vi "SUNSoftwareBinCheckReceivedQty.vi"() -> ()   [LabVIEW 2012]
uses:
  <vilib>/addons/database/Auxilliary.llb/DB Tools Cursor Type.ctl
  <vilib>/Utility/NIReport.llb/NI_report.lvclass
  <vilib>/addons/database/Connection.llb/DB Tools Open Connec (Path).vi
  <vilib>/addons/database/Connection.llb/Conn Execute.vi
  <vilib>/addons/database/Recordset.llb/Rec Fetch Recordset Data (R).vi
  <vilib>/addons/database/Recordset.llb/Rec Destroy - Connection.vi
  <vilib>/addons/database/Recordset.llb/Rec Fetch Integer Data (R).vi
  <vilib>/Utility/NIReport.llb/Append Text Table to Report (wrap).vi
  <vilib>/addons/database/_DB Variant To Data/Database Variant To Data.xnode
  <vilib>/addons/database/NI_Database_API.lvlib
  <vilib>/Utility/NIReport.llb/Excel/NI_Excel.lvclass
panel:
  out "recordset data":variant[][](array[variant])
  out "data":string
  out "appended array":string[](array[string])
  out "concatenated string":string
  in  "Report Template":path=path "O:/Monitor/Report/MSTsoftBin.xls"
  out "Row Headers":string[](array[string])
  out "error out 2":errorcluster
  out "error out":errorcluster
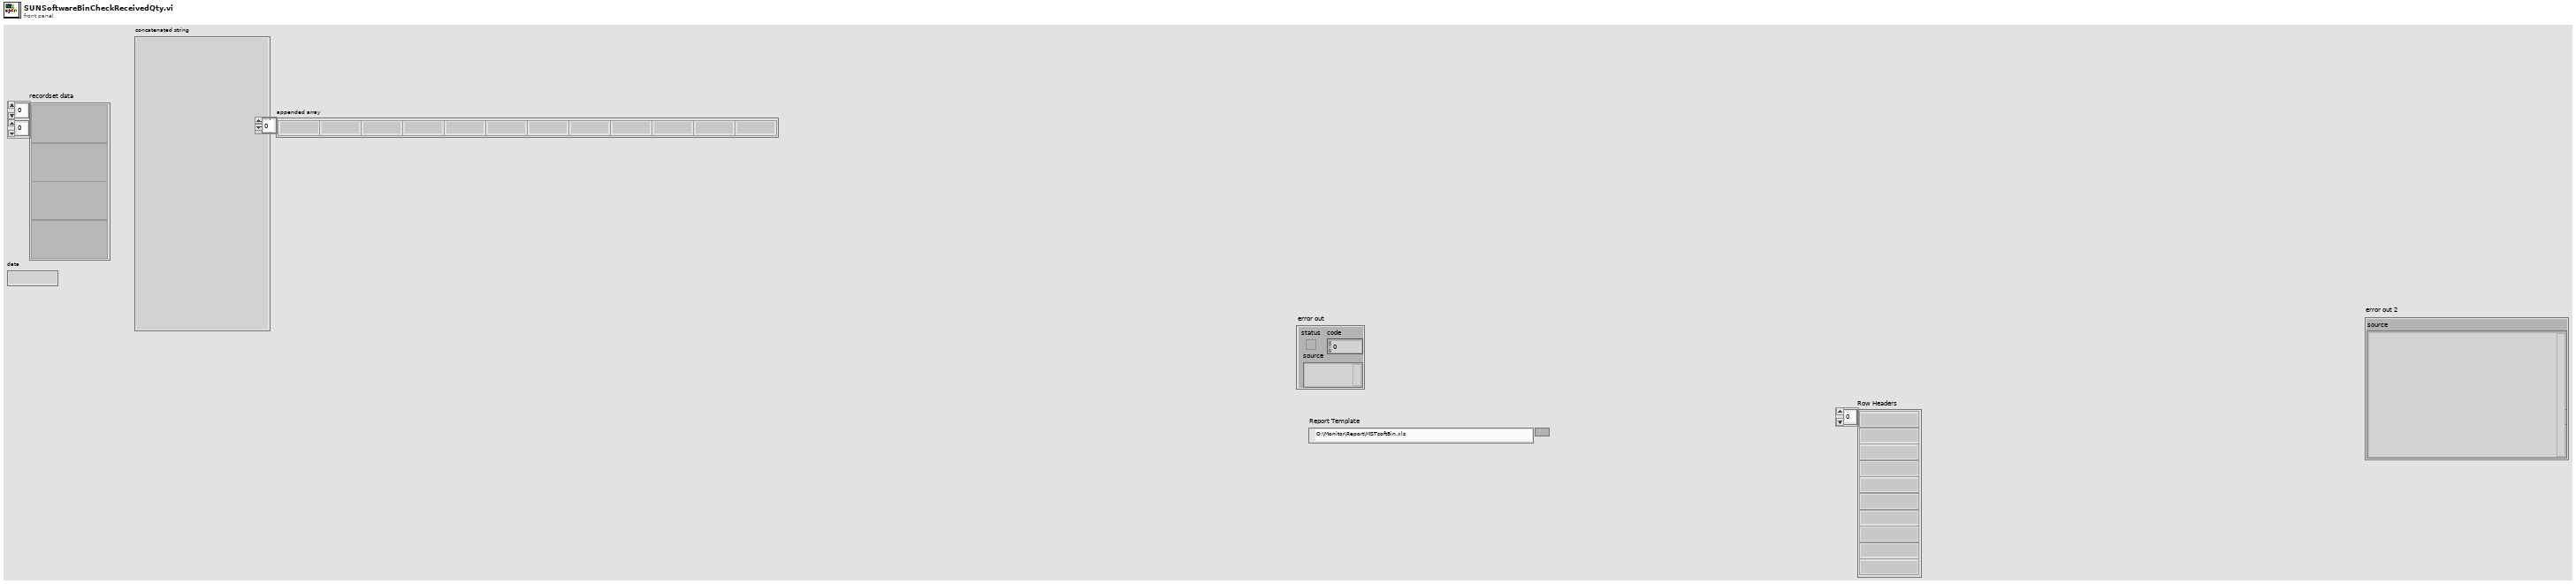
[diagram p1: front panel]
types:
  T1 = typedef "NI_Database_API.lvlib/DB Tools Cursor Type.ctl" = enum16{"forward-only", "keyset", "dynamic", "static"}
  T2 = enum16{"Standard Report", "HTML", "Word", "Excel"}
  T3 = typedef "NI_Database_API.lvlib/Conn ObjectReference.ctl" = refnum<k1>
  T4 = typedef "NI_Database_API.lvlib/Rec ObjectReference.ctl" = refnum<k1>
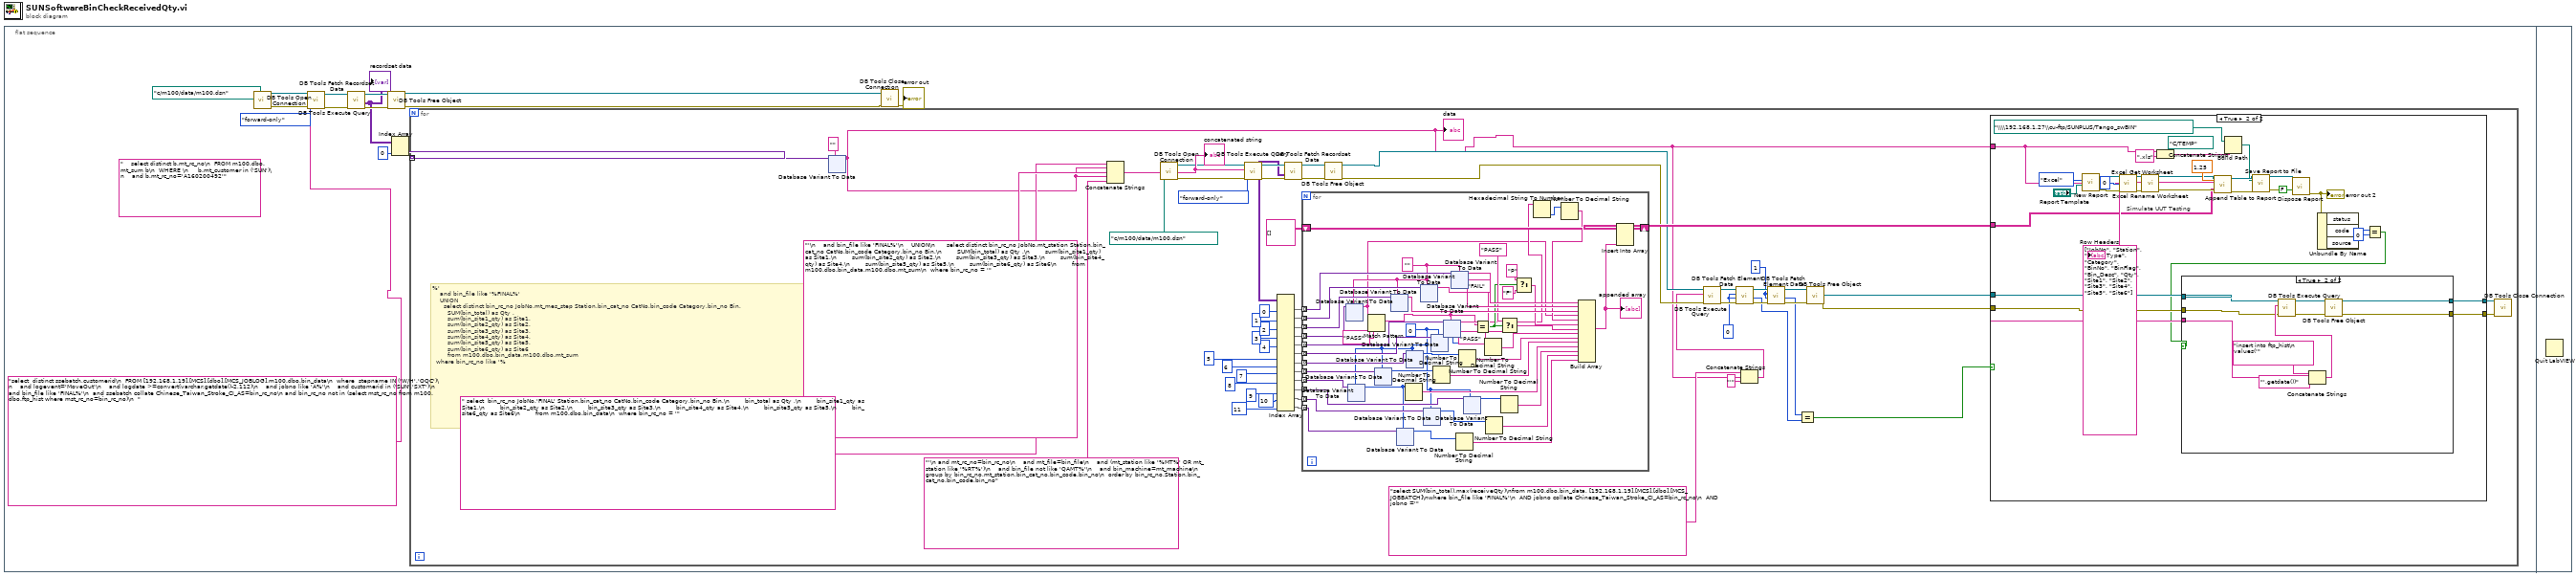
[diagram p0: block diagram]
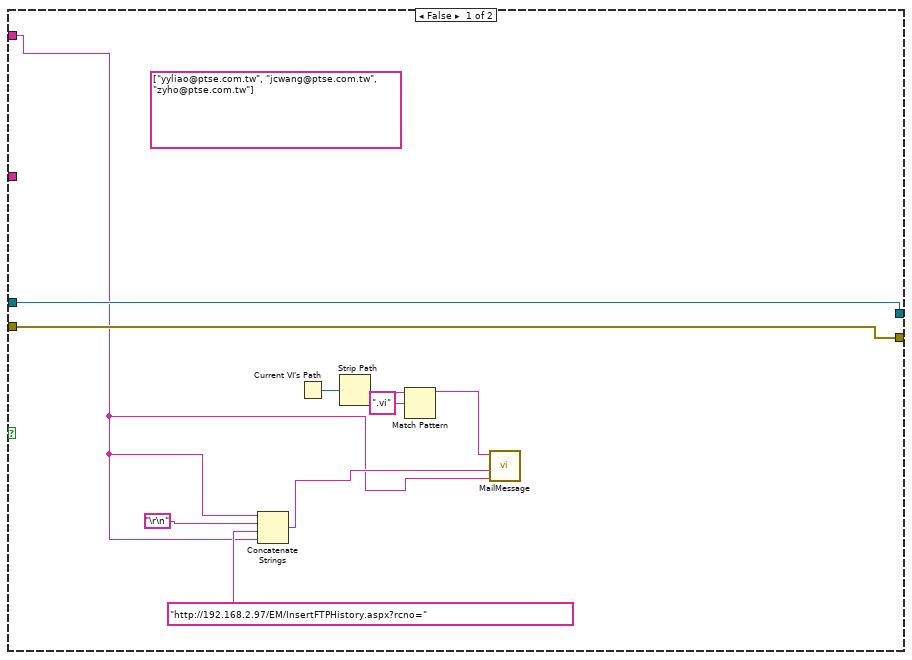
[diagram p2: hidden frame]
diagram:
  n1 = flat-sequence {
    frame #0 {
      (unwired) "    select distinct b.mt_rc_no\n  FROM m100.dbo.mt_sum b\n  WHERE \n     b.mt_customer in ('SUN')\n    and b.mt_rc_no='A160200492'" ("SQL query")
      n2 = call-poly <vilib>:"DB Tools Open Connection.vi"("connection information"=path "c:/m100/data/m100.dsn") -> ("error out"=w12:errorcluster, "connection reference"=w15:T3)  [unwired: 7 in]
      n3 = call-poly <vilib>:"DB Tools Execute Query.vi"("error in (no error)"=w12, "cursor type"=DB_Tools_Cursor_Type."forward-only", "SQL query"="select  distinct ssebatch,customerid\n  FROM [192.168.1.19].[MCS].[dbo].[MCS_JOBLOG],m100.dbo.bin_data\n  where  stepname IN ('W/H','OQC')\n    and logevent='MoveOut'\n    and logdate >=convert(varchar,getdate()-2,112)\n    and jobno like 'A%'\n    and customerid in ('SUN','SXT')\n  and bin_file like 'FINAL%'\n  and ssebatch collate Chinese_Taiwan_Stroke_CI_AS=bin_rc_no\n and bin_rc_no not in (select mst_rc_no from m100.dbo.ftp_hist where mst_rc_no=bin_rc_no)\n  ", "connection reference"=w15) -> ("error out"=w11:errorcluster, "recordset reference"=w14:T4)  [unwired: 4 in]
      n4 = call-poly <vilib>:"DB Tools Fetch Recordset Data.vi"("error in (no error)"=w11, "recordset reference"=w14) -> ("error out"=w10:errorcluster, "recordset data"=w7:variant[][], "recordset reference out"=w13:T4)  [unwired: 3 in]
      "recordset data" <- w7
      n5 = call-poly <vilib>:"DB Tools Free Object.vi"("error in (no error)"=w10, "recordset reference"=w13) -> ("error out"=w3:errorcluster, "connection reference"=w4:T3)  [unwired: 8 in]
      n6 = Index Array(array=w7, index (col)=0 ("disabled index (col)")) -> (element=w5:variant[])  [unwired: 1 in]
      n7 = for {
        tunnel: w5 -> [w77] mode=indexing
        w21 = 1
        w22 = 0
        # "%'\n    and bin_file like '%FINAL%'\n    UNION\n      select distinct bin_rc_no JobNo,mt_mes_step Station,bin_cat_no CatNo,bin_code Category,bin_no Bin,\n        SUM(bin_total) as Qty ,\n        sum(bin_site1_qty) as Site1,\n        sum(bin_site2_qty) as Site2,\n        sum(bin_site3_qty) as Site3,\n        sum(bin_site4_qty) as Site4,\n        sum(bin_site5_qty) as Site5,\n        sum(bin_site6_qty) as Site6\n        from m100.dbo.bin_data,m100.dbo.mt_sum\n  where bin_rc_no like '%"
        n8 = xnode "Database Variant To Data"("database variant"=w77, "type"="") -> ("data"=w25:string)  [unwired: 1 in, 1 out]
        "data" <- w25
        n9 = Concatenate Strings(" select  bin_rc_no JobNo,'FINAL' Station,bin_cat_no CatNo,bin_code Category,bin_no Bin,\n        bin_total as Qty ,\n        bin_site1_qty as Site1,\n        bin_site2_qty as Site2,\n        bin_site3_qty as Site3,\n        bin_site4_qty as Site4,\n        bin_site5_qty as Site5,\n        bin_site6_qty as Site6\n        from m100.dbo.bin_data\n  where bin_rc_no = '" ("string"), w25, "'\n    and bin_file like 'FINAL%'\n    UNION\n      select distinct bin_rc_no JobNo,mt_station Station,bin_cat_no CatNo,bin_code Category,bin_no Bin,\n        SUM(bin_total) as Qty ,\n        sum(bin_site1_qty) as Site1,\n        sum(bin_site2_qty) as Site2,\n        sum(bin_site3_qty) as Site3,\n        sum(bin_site4_qty) as Site4,\n        sum(bin_site5_qty) as Site5,\n        sum(bin_site6_qty) as Site6\n        from m100.dbo.bin_data,m100.dbo.mt_sum\n  where bin_rc_no = '" ("string"), w25, "'\n and mt_rc_no=bin_rc_no\n    and mt_file=bin_file\n    and (mt_station like '%MT%' OR mt_station like '%RT%')\n    and bin_file not like 'QAMT%'\n    and bin_machine=mt_machine\n  group by bin_rc_no,mt_station,bin_cat_no,bin_code,bin_no\n  order by bin_rc_no,Station,bin_cat_no,bin_code,bin_no" ("string")) -> (w68:string)
        "concatenated string" <- w68
        n10 = call-poly <vilib>:"DB Tools Open Connection.vi"("connection information"=path "c:/m100/data/m100.dsn") -> ("error out"=w39:errorcluster, "connection reference"=w40:T3)  [unwired: 7 in]
        n11 = call-poly <vilib>:"DB Tools Execute Query.vi"("error in (no error)"=w39, "cursor type"=DB_Tools_Cursor_Type."forward-only", "SQL query"=w68, "connection reference"=w40) -> ("error out"=w73:errorcluster, "recordset reference"=w75:T4)  [unwired: 4 in]
        n12 = call-poly <vilib>:"DB Tools Fetch Recordset Data.vi"("error in (no error)"=w73, "recordset reference"=w75) -> ("error out"=w72:errorcluster, "recordset data"=w67:variant[][], "recordset reference out"=w74:T4)  [unwired: 3 in]
        n13 = Index Array(array=w67, index (col) #1=0 ("disabled index (col)"), index (col) #2=1 ("index (col)"), index (col) #3=2 ("index (col)"), index (col) #4=3 ("index (col)"), index (col) #5=4 ("index (col)"), index (col) #6=5 ("index (col)"), index (col) #7=6 ("index (col)"), index (col) #8=7 ("index (col)"), index (col) #9=8 ("index (col)"), index (col) #10=9 ("index (col)"), index (col) #11=10 ("index (col)"), index (col) #12=11 ("index (col)")) -> (element #1=w56:variant[], element #2=w55:variant[], element #3=w54:variant[], element #4=w53:variant[], element #5=w52:variant[], element #6=w51:variant[], element #7=w50:variant[], element #8=w49:variant[], element #9=w48:variant[], element #10=w47:variant[], element #11=w44:variant[], element #12=w43:variant[])  [unwired: 12 in]
        n14 = for {
          tunnel: w56 -> [w177] mode=indexing
          tunnel: w55 -> [w176] mode=indexing
          tunnel: w54 -> [w175] mode=indexing
          tunnel: w53 -> [w174] mode=indexing
          tunnel: w52 -> [w173] mode=indexing
          tunnel: w51 -> [w172] mode=indexing
          tunnel: w50 -> [w171] mode=indexing
          tunnel: w49 -> [w170] mode=indexing
          tunnel: w48 -> [w169] mode=indexing
          tunnel: w47 -> [w168] mode=indexing
          tunnel: w44 -> [w159] mode=indexing
          tunnel: w43 -> [w158] mode=indexing
          shift-right: [w153] -> w41
          shift-left: string[][] [] ("array") -> [w152]
          w144 = 0
          w167 = ""
          n15 = xnode "Database Variant To Data"("database variant"=w174, "type"=w167) -> ("data"=w132:string)  [unwired: 1 in, 1 out]
          n16 = xnode "Database Variant To Data"("database variant"=w169, "type"=w144) -> ("data"=w156:i32)  [unwired: 1 in, 1 out]
          n17 = Match Pattern(string=w132, regular expression="PASS") -> (match substring=w130:string)  [unwired: 1 in, 3 out]
          n18 = xnode "Database Variant To Data"("database variant"=w170, "type"=w144) -> ("data"=w161:i32)  [unwired: 1 in, 1 out]
          n19 = xnode "Database Variant To Data"("database variant"=w175, "type"=w167) -> ("data"=w164:string)  [unwired: 1 in, 1 out]
          n20 = xnode "Database Variant To Data"("database variant"=w158, "type"=w156) -> ("data"=w157:i32)  [unwired: 1 in, 1 out]
          n21 = Number To Decimal String(number=w156) -> (decimal integer string=w148:string)  [unwired: 1 in]
          n22 = xnode "Database Variant To Data"("database variant"=w171, "type"=w144) -> ("data"=w162:i32)  [unwired: 1 in, 1 out]
          n23 = xnode "Database Variant To Data"("database variant"=w176, "type"=w167) -> ("data"=w165:string)  [unwired: 1 in, 1 out]
          n24 = xnode "Database Variant To Data"("database variant"=w159, "type"=w144) -> ("data"=w155:i32)  [unwired: 1 in, 1 out]
          n25 = xnode "Database Variant To Data"("database variant"=w172, "type"=w144) -> ("data"=w163:i32)  [unwired: 1 in, 1 out]
          n26 = Number To Decimal String(number=w161) -> (decimal integer string=w147:string)  [unwired: 1 in]
          n27 = xnode "Database Variant To Data"("database variant"=w173, "type"=w130) -> ("data"=w134:string)  [unwired: 1 in, 1 out]
          n28 = xnode "Database Variant To Data"("database variant"=w177, "type"=w167) -> ("data"=w166:string)  [unwired: 1 in, 1 out]
          n29 = Number To Decimal String(number=w157) -> (decimal integer string=w151:string)  [unwired: 1 in]
          n30 = Number To Decimal String(number=w162) -> (decimal integer string=w146:string)  [unwired: 1 in]
          n31 = xnode "Database Variant To Data"("database variant"=w168, "type"=w144) -> ("data"=w160:i32)  [unwired: 1 in, 1 out]
          n32 = Equal?(x=w130, y="PASS") -> (x = y?=w140:bool)
          n33 = Number To Decimal String(number=w163) -> (decimal integer string=w145:string)  [unwired: 1 in]
          n34 = Number To Decimal String(number=w155) -> (decimal integer string=w150:string)  [unwired: 1 in]
          n35 = Number To Decimal String(number=w160) -> (decimal integer string=w149:string)  [unwired: 1 in]
          n36 = Select(t="PASS", s=w140, f="FAIL") -> (s? t:f=w141:string)
          n37 = Select(t="P", s=w140, f="F") -> (s? t:f=w137:string)
          n38 = Hexadecimal String To Number(string=w134) -> (number=w135:u32)  [unwired: 2 in, 1 out]
          n39 = Number To Decimal String(number=w135) -> (decimal integer string=w133:string)  [unwired: 1 in]
          n40 = Build Array(w166, w165, w164, w132, w133, w137, w141, w145, w146, w147, w148, w149, w150, w151) -> (w154:string[])
          "appended array" <- w154
          n41 = Insert Into Array(array=w152, new element=w154) -> (w153:string[][])  [unwired: 2 in]
        }
        n42 = call-poly <vilib>:"DB Tools Free Object.vi"("error in (no error)"=w72, "recordset reference"=w74) -> ("error out"=w35:errorcluster, "connection reference"=w36:T3)  [unwired: 8 in]
        n43 = Concatenate Strings("select SUM(bin_total),max(receiveQty)\nfrom m100.dbo.bin_data, [192.168.1.19].[MCS].[dbo].[MCS_JOBBATCH]\nwhere bin_file like 'FINAL%'\n  AND jobno collate Chinese_Taiwan_Stroke_CI_AS=bin_rc_no\n  AND jobno ='" ("SQL query"), w25, "'" ("string")) -> (w23:string)
        n44 = call-poly <vilib>:"DB Tools Execute Query.vi"("error in (no error)"=w35, "SQL query"=w23, "connection reference"=w36) -> ("error out"=w33:errorcluster, "recordset reference"=w34:T4)  [unwired: 5 in]
        n45 = call-poly <vilib>:"DB Tools Fetch Element Data.vi"("error in (no error)"=w33, "type"=w22, "column index"=w22, "recordset reference"=w34) -> ("error out"=w31:errorcluster, "data"=w19:i32, "recordset reference out"=w32:T4)  [unwired: 3 in]
        n46 = call-poly <vilib>:"DB Tools Fetch Element Data.vi"("error in (no error)"=w31, "type"=w21, "column index"=w21, "recordset reference"=w32) -> ("error out"=w29:errorcluster, "data"=w20:i32, "recordset reference out"=w30:T4)  [unwired: 3 in]
        n47 = Equal?(x=w20, y=w19) -> (x = y?=w16:bool)
        n48 = call-poly <vilib>:"DB Tools Free Object.vi"("error in (no error)"=w29, "recordset reference"=w30) -> ("error out"=w27:errorcluster, "connection reference"=w28:T3)  [unwired: 8 in]
        n49 = case shown="True" w16 {
          tunnel: w41 -> [_ w106]
          tunnel: w28 -> [w87 w93]
          tunnel: w27 -> [w86 w92]
          tunnel: w25 -> [w78 w91]
          tunnel: [w87 w89] -> w18
          tunnel: [w86 w88] -> w17
          frame False {
            (unwired) string[] ["yyliao@ptse.com.tw", "jcwang@ptse.com.tw", "zyho@ptse.com.tw"] ("recipients")
            n50 = Concatenate Strings(w78, "\r\n", "http://192.168.2.97/EM/InsertFTPHistory.aspx?rcno=" ("string"), w78) -> (w79:string)
            n51 = Current VI's Path() -> (path=w83:path)
            n52 = Strip Path(path=w83) -> (name=w82:string)  [unwired: 1 out]
            n53 = Match Pattern(string=w82, regular expression=".vi") -> (before substring=w80:string)  [unwired: 1 in, 3 out]
            n54 = call "MailMessage.vi"("AddSubject"=w78, "message"=w79, "program"=w80) -> ()  [unwired: 9 in]
          }
          frame True {
            (unwired) path "C:/TEMP" ("base path")
            # "Simulate UUT Testing"
            n55 = call <vilib>:"New Report.vi"("report type"=T2."Excel" ("Report Type"), "template (empty)"="Report Template") -> ("report out"=w113:refnum<class "NI_report.lvclass">, "error out"=w112:errorcluster)  [unwired: 12 in]
            n56 = call <vilib>:"Excel Get Worksheet.vi"("report in"=w113, "worksheet index (0)"=0, "error in (no error)"=w112) -> ("report out"=w110:refnum<class "NI_report.lvclass">, "error out"=w108:errorcluster)  [unwired: 11 in]
            n57 = call <vilib>:"Excel Rename Worksheet.vi"("report in"=w110, "worksheet name (\"\")"=w91, "error in (no error)"=w108) -> ("report out"=w109:refnum<class "NI_report.lvclass">, "error out"=w107:errorcluster)  [unwired: 11 in]
            n58 = Concatenate Strings(w91, ".xls" ("string")) -> (w99:string)
            n59 = call-poly <vilib>:"Append Table to Report.vi"("report in"=w109, "column width (1)"=1.25, "column headers"=string[] ["JobNo", "Station", "CatNo Type", "Category", "BinNo", "BinFlag", "Bin_Desc", "Qty", "Site1", "Site2", "Site3", "Site4", "Site5", "Site6"] ("row headers"), "text data"=w106, "error in (no error)"=w107) -> ("report out"=w102:refnum<class "NI_report.lvclass">, "error out"=w101:errorcluster)  [unwired: 7 in, 2 out]
            n60 = Build Path(base path=path "\\\\192.168.1.27\\cu-ftp/SUNPLUS/Tango_swBIN", name or relative path=w99) -> (appended path=w98:path)
            n61 = call-dynamic "Save Report to File.vi"("report in"=w102, "report file path"=w98, "error in (no error)"=w101) -> ("report out"=w104:refnum<class "NI_report.lvclass">, "error out"=w103:errorcluster)  [unwired: 11 in]
            n62 = call-dynamic "Dispose Report.vi"("report in"=w104, "save changes? (F)"=FALSE, "error in (no error)"=w103) -> ("error out"=w97:errorcluster)  [unwired: 12 in]
            "error out 2" <- w97
            n63 = Unbundle By Name(w97) -> ("code"=w96:i32)  [unwired: 2 out]
            n64 = Equal?(x=w96, y=0) -> (x = y?=w90:bool)
            n65 = case shown="True" w90 {
              tunnel: w93 -> [w119 w129]
              tunnel: w91 -> [_ w127]
              tunnel: [w119 w122] -> w89
              tunnel: [w118 w121] -> w88
              tunnel: w92 -> [w118 w120]
              frame False {
              }
              frame True {
                n66 = Concatenate Strings("insert into ftp_hist\n values('" ("string"), w127, "',getdate())" ("string")) -> (w125:string)
                n67 = call-poly <vilib>:"DB Tools Execute Query.vi"("error in (no error)"=w120, "SQL query"=w125, "connection reference"=w129) -> ("error out"=w123:errorcluster, "recordset reference"=w124:T4)  [unwired: 5 in]
                n68 = call-poly <vilib>:"DB Tools Free Object.vi"("error in (no error)"=w123, "recordset reference"=w124) -> ("error out"=w121:errorcluster, "connection reference"=w122:T3)  [unwired: 8 in]
              }
            }
          }
        }
        n69 = call <vilib>:"DB Tools Close Connection.vi"("error in (no error)"=w17, "connection reference"=w18) -> ()  [unwired: 5 in, 1 out]
      }
      n70 = call <vilib>:"DB Tools Close Connection.vi"("error in (no error)"=w3, "connection reference"=w4) -> ("error out"=→"error out":errorcluster)  [unwired: 5 in]
    }
    frame #1 {
      n71 = Quit LabVIEW() -> ()  [unwired: 1 in]
    }
  }
